vi "ir read test 3.vi"   [LabVIEW 2012, in "BlockParty4150.lvrbt"]
uses:
  BlockParty4150.lvrbt
  <vilib>/NXT/HiTechnic/HiTechnic Controls/HiTechnic Port.ctl
  <vilib>/NXT/Block Support/NXT_InputPort.ctl
types:
  T1 = typedef "HiTechnic Port.ctl" = cluster{"Port":T2, "MUX Port":u8}
  T2 = typedef "NXT_InputPort.ctl" = u8
  T3 = cluster{"Direction (0-9)":i16, "Signal Strength (Array)":u8[]}
  T4 = typedef "LVHSConnector.ctl" = refnum<class "BrickReference.lvclass">
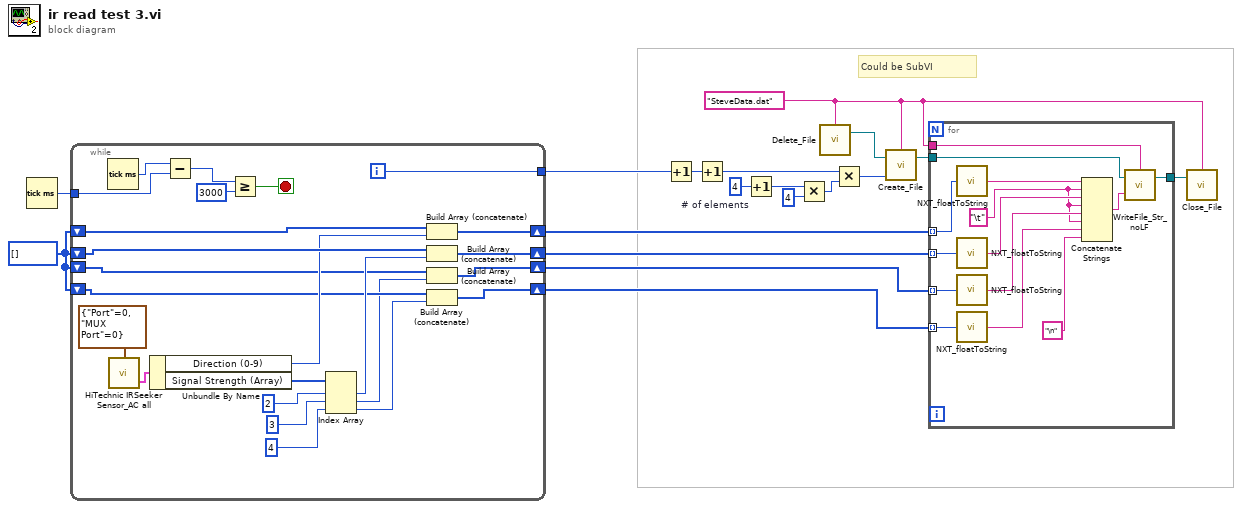
[diagram p0: block diagram]
diagram:
  w3 = u32[] []
  w12 = 4  # # of elements
  w8 = "SteveData.dat" ("Filename")
  # "Could be SubVI"
  n1 = Tick Count (ms)() -> (millisecond timer value=w18:u32)
  n2 = while {
    tunnel: w18 -> [w41]
    tunnel: [w38] -> w10
    shift-right: [w37] -> w6
    shift-left: w3 -> [w36]
    shift-right: [w33] -> w5
    shift-left: w3 -> [w34]
    shift-right: [w20] -> w2
    shift-left: w3 -> [w24]
    shift-right: [w19] -> w1
    shift-left: w3 -> [w23]
    i -> [w38]
    stop <- w39 stop-if-true
    n3 = Tick Count (ms)() -> (millisecond timer value=w42:u32)
    n4 = call <vilib>:"HiTechnic IRSeeker Sensor_AC all.vi"("Port/MUX"=T1 {"Port"=0, "MUX Port"=0}) -> ("All Info"=w32:T3)  [unwired: 2 in, 1 out]
    n5 = Unbundle By Name(w32) -> ("Direction (0-9)"=w27:i16, "Signal Strength (Array)"=w31:u8[])
    n6 = Subtract(x=w42, y=w41) -> (x-y=w35:u32)
    n7 = Greater Or Equal?(x=w35, y=u32 3000) -> (x >= y?=w39:bool)
    n8 = Index Array(array=w31, index #1=2 ("index"), index #2=3 ("index"), index #3=4 ("index")) -> (element #1=w29:u8, element #2=w22:u8, element #3=w21:u8)
    n9 = Build Array (concatenate)(w36, w27) -> (w37:u32[])
    n10 = Build Array (concatenate)(w34, w29) -> (w33:u32[])
    n11 = Build Array (concatenate)(w24, w22) -> (w20:u32[])
    n12 = Build Array (concatenate)(w23, w21) -> (w19:u32[])
  }
  n13 = Increment(x=w10) -> (x+1=w9:i32)
  n14 = Increment(x=w9) -> (x+1=w16:i32)
  n15 = Increment(x=w12) -> (x+1=w13:i32)
  n16 = Multiply(x=w13, y=u32 4) -> (x*y=w14:u32)
  n17 = call <vilib>:"Delete_File.vi"("Filename"=w8) -> ("NXT"=w17:T4)  [unwired: 3 in]
  n18 = Multiply(x=w16, y=w14) -> (x*y=w4:u32)
  n19 = call <vilib>:"Create_File.vi"("File Size (256)"=w4, "NXT"=w17, "Filename"=w8) -> ("NXT"=w7:T4)  [unwired: 1 out]
  n20 = for {
    tunnel: w8 -> [w56]
    tunnel: w7 -> [w55]
    tunnel: [w54] -> w11
    tunnel: w6 -> [w53] mode=indexing
    tunnel: w5 -> [w51] mode=indexing
    tunnel: w2 -> [w44] mode=indexing
    tunnel: w1 -> [w43] mode=indexing
    w47 = "\t" ("string")
    n21 = call <vilib>:"NXT_floatToString.vi"("number"=w53) -> ("string"=w50:string)
    n22 = call <vilib>:"NXT_floatToString.vi"("number"=w51) -> ("string"=w49:string)
    n23 = call <vilib>:"NXT_floatToString.vi"("number"=w44) -> ("string"=w48:string)
    n24 = call <vilib>:"NXT_floatToString.vi"("number"=w43) -> ("string"=w46:string)
    n25 = Concatenate Strings(w50, w47, w49, w47, w48, w47, w46, "\n") -> (w52:string)
    n26 = call <vilib>:"WriteFile_Str_noLF.vi"("String"=w52, "NXT"=w55, "Filename"=w56) -> ("NXT"=w54:T4)  [unwired: 1 in]
  }
  n27 = call <vilib>:"Close_File.vi"("NXT"=w11, "Filename"=w8) -> ()  [unwired: 2 in, 1 out]
